vi "Servo MSMT TDSCDMA Configure Measure Step.vi"(8 "error in (no error)":errorcluster, 11 "Servo MSMT in":refnum<class "Servo MSMT.lvclass">) -> (0 "error out":errorcluster, 3 "Servo MSMT out":refnum<class "Servo MSMT.lvclass">)   [LabVIEW 2018, in "Servo MSMT.lvlib" / "Servo MSMT.lvclass"]
uses:
  Servo MSMT.lvclass
  C:/Sequence Automation/Plugins/Measurement Interface.lvlibp/Measurement Interface.lvclass
  Plugins/Measurement Interface.lvlibp/Private Methods/Measurement Name/Read Measurement Name.vi
  Plugins/TestStand API Tools (TSAT).lvlibp/Step Actions/TSAT Step Actions.lvlib
  Plugins/Measurement Interface.lvlibp/Measurement Interface.lvclass
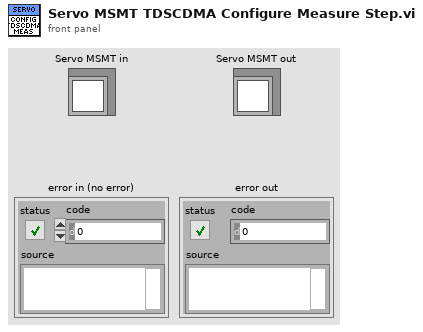
[diagram p1: front panel]
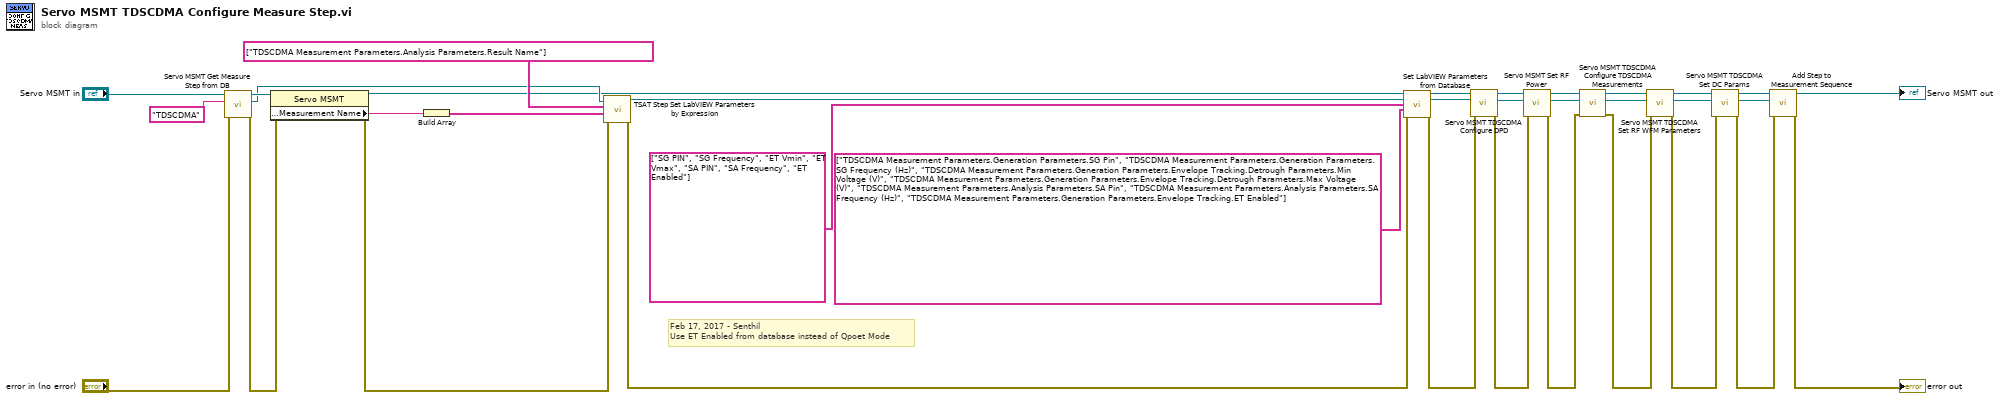
[diagram p0: block diagram]
diagram:
  # "Feb 17, 2017 - Senthil\nUse ET Enabled from database instead of Qpoet Mode"
  n1 = call "Servo MSMT Get Measure Step from DB.vi"("error in (no error)"="error in (no error)", "Standard"="TDSCDMA", "Servo MSMT in"="Servo MSMT in") -> ("error out"=w17:errorcluster, "Step Out"=w20:refnum<k7>, "Servo MSMT out"=w22:refnum<class "Servo MSMT.lvclass">)  [unwired: 6 in]
  n2 = property class="Servo MSMT"(reference=w22, error in=w17) -> (reference out=w1:refnum<class "Servo MSMT.lvclass">, error out=w16:errorcluster, "Public Methods:Measurement Name"=w19:string)
  n3 = Build Array(w19) -> (w35:string[])
  n4 = call "TSAT Step Set LabVIEW Parameters by Expression.vi"("Error In"=w16, "Value Expressions"=w35, "Parameters to Set"=string[] ["TDSCDMA Measurement Parameters.Analysis Parameters.Result Name"], "Step In"=w20) -> ("Error Out"=w33:errorcluster, "Step Out"=w2:refnum<k7>)  [unwired: 6 in]
  n5 = call "Set LabVIEW Parameters from Database.vi"("Measurement Interface in"=w1, "Step In"=w2, "Dictionary Keys"=string[] ["SG PIN", "SG Frequency", "ET Vmin", "ET Vmax", "SA PIN", "SA Frequency", "ET Enabled"] ("Database Keys"), "LabVIEW Parameter Mapping"=string[] ["TDSCDMA Measurement Parameters.Generation Parameters.SG Pin", "TDSCDMA Measurement Parameters.Generation Parameters.SG Frequency (Hz)", "TDSCDMA Measurement Parameters.Generation Parameters.Envelope Tracking.Detrough Parameters.Min Voltage (V)", "TDSCDMA Measurement Parameters.Generation Parameters.Envelope Tracking.Detrough Parameters.Max Voltage (V)", "TDSCDMA Measurement Parameters.Analysis Parameters.SA Pin", "TDSCDMA Measurement Parameters.Analysis Parameters.SA Frequency (Hz)", "TDSCDMA Measurement Parameters.Generation Parameters.Envelope Tracking.ET Enabled"] ("Database Keys"), "error in (no error)"=w33) -> ("Measurement Interface out"=w11:refnum<class "Servo MSMT.lvclass">, "Step Out"=w9:refnum<k7>, "error out"=w14:errorcluster)  [unwired: 8 in]
  n6 = call "Servo MSMT TDSCDMA Configure DPD.vi"("error in (no error)"=w14, "Step In"=w9, "Servo MSMT in"=w11) -> ("error out"=w12:errorcluster, "Step Out"=w8:refnum<k7>, "Servo MSMT out"=w10:refnum<class "Servo MSMT.lvclass">)  [unwired: 6 in]
  n7 = call-dynamic "Servo MSMT Set RF Power.vi"("error in (no error)"=w12, "Step In"=w8, "Servo MSMT in"=w10) -> ("error out"=w4:errorcluster, "Step Out"=w6:refnum<k7>, "Servo MSMT out"=w15:refnum<class "Servo MSMT.lvclass">)  [unwired: 6 in]
  n8 = call "Servo MSMT TDSCDMA Configure TDSCDMA Measurements.vi"("error in (no error)"=w4, "Step In"=w6, "Servo MSMT in"=w15) -> ("error out"=w3:errorcluster, "Step Out"=w5:refnum<k7>, "Servo MSMT out"=w7:refnum<class "Servo MSMT.lvclass">)  [unwired: 6 in]
  n9 = call "Servo MSMT TDSCDMA Set RF WFM Parameters.vi"("error in (no error)"=w3, "Step In"=w5, "Servo MSMT in"=w7) -> ("error out"=w27:errorcluster, "Step Out"=w24:refnum<k7>, "Servo MSMT out"=w29:refnum<class "Servo MSMT.lvclass">)  [unwired: 6 in]
  n10 = call "Servo MSMT TDSCDMA Set DC Params.vi"("error in (no error)"=w27, "Step In"=w24, "Servo MSMT in"=w29) -> ("error out"=w28:errorcluster, "Step Out"=w23:refnum<k7>, "Servo MSMT out"=w31:refnum<class "Servo MSMT.lvclass">)  [unwired: 6 in]
  n11 = call "Add Step to Measurement Sequence.vi"("error in (no error)"=w28, "Step to Add"=w23, "Measurement Interface in"=w31) -> ("error out"=→"error out":errorcluster, "Measurement Interface out"=→"Servo MSMT out":refnum<class "Servo MSMT.lvclass">)  [unwired: 7 in]
